vi "S4GUI.vi"(7 "Tab ObsEng":enum32{"Obs", "CCD modes", "Eng"}(tab)) -> ()   [LabVIEW 2018] (continued)
            n3007 = call-dynamic "Write State Machine.vi"("error in (no error)"=w6568, "State Machine.lvclass"=w6572, "Device in"=w6570) -> ("error out"=w6574:errorcluster, "Device out"=w6573:refnum<class "Channel.lvclass">)  [unwired: 7 in]
            n3008 = call-dynamic "Write Channel.vi"("error in (no error)"=w6574, "Channel.lvclass"=w6573, "Acquisition in"=w6566) -> ("error out"=w6562:errorcluster, "Acquisition out"=w6563:refnum<class "Acquisition.lvclass">)  [unwired: 7 in]
          }
        }
        n3009 = case shown="True" w6446 {
          tunnel: w6448 -> [w6490 w6522]
          tunnel: w6447 -> [w6489 w6521]
          tunnel: [w6490 w6520] -> w6469
          tunnel: [w6489 w6519] -> w6468
          tunnel: w6459 -> [_ w6502]
          tunnel: w6433 -> [_ w6501]
          tunnel: w6434 -> [_ w6500]
          tunnel: w6427 -> [_ w6499]
          tunnel: w6432 -> [_ w6498]
          tunnel: w6431 -> [_ w6493]
          frame False {
          }
          frame True {
            (unwired) 12 ("State")
            n3010 = call-dynamic "Read Channel.vi"("error in (no error)"=w6521, "Acquisition in"=w6522) -> ("error out"=w6496:errorcluster, "Channel.lvclass"=w6497:refnum<class "Channel.lvclass">, "Acquisition out"=w6531:refnum<class "Acquisition.lvclass">)  [unwired: 7 in]
            n3011 = local read "Filter4"() -> (w6503:u8)
            n3012 = call-dynamic "Write Filter.vi"("error in (no error)"=w6496, "Filter"=w6503, "Channel in"=w6497) -> ("error out"=w6518:errorcluster, "Channel out"=w6507:refnum<class "Channel.lvclass">)  [unwired: 7 in]
            n3013 = call-dynamic "Read Interface.vi"("error in (no error)"=w6518, "Channel in"=w6507) -> ("error out"=w6517:errorcluster, "Interface.lvclass"=w6516:refnum<class "Interface.lvclass">, "Channel out"=w6506:refnum<class "Channel.lvclass">)  [unwired: 7 in]
            n3014 = call-dynamic "Write Suffix.vi"("error in (no error)"=w6517, "Suffix"=w6502, "Interface in"=w6516) -> ("error out"=w6508:errorcluster, "Interface out"=w6511:refnum<class "Interface.lvclass">)  [unwired: 7 in]
            n3015 = call-dynamic "Write ObsType.vi"("error in (no error)"=w6508, "ObsType"=w6501, "Interface in"=w6511) -> ("error out"=w6509:errorcluster, "Interface out"=w6512:refnum<class "Interface.lvclass">)  [unwired: 7 in]
            n3016 = call-dynamic "Write Object.vi"("error in (no error)"=w6509, "Object"=w6500, "Interface in"=w6512) -> ("error out"=w6510:errorcluster, "Interface out"=w6513:refnum<class "Interface.lvclass">)  [unwired: 7 in]
            n3017 = call-dynamic "Write Comments.vi"("error in (no error)"=w6510, "Comments"=w6499, "Interface in"=w6513) -> ("error out"=w6514:errorcluster, "Interface out"=w6515:refnum<class "Interface.lvclass">)  [unwired: 7 in]
            n3018 = call-dynamic "Write Observer.vi"("error in (no error)"=w6514, "Observer"=w6498, "Interface in"=w6515) -> ("error out"=w6495:errorcluster, "Interface out"=w6494:refnum<class "Interface.lvclass">)  [unwired: 7 in]
            n3019 = call-dynamic "Write Project ID.vi"("error in (no error)"=w6495, "Project ID"=w6493, "Interface in"=w6494) -> ("error out"=w6491:errorcluster, "Interface out"=w6492:refnum<class "Interface.lvclass">)  [unwired: 7 in]
            n3020 = call-dynamic "Write Interface.vi"("error in (no error)"=w6491, "Interface.lvclass"=w6492, "Channel in"=w6506) -> ("error out"=w6504:errorcluster, "Channel out"=w6505:refnum<class "Channel.lvclass">)  [unwired: 7 in]
            n3021 = call-dynamic "Read State Machine.vi"("error in (no error)"=w6504, "Device in"=w6505) -> ("error out"=w6530:errorcluster, "State Machine.lvclass"=w6526:refnum<class "State Machine.lvclass">, "Device out"=w6527:refnum<class "Channel.lvclass">)  [unwired: 7 in]
            n3022 = call-dynamic "Write State.vi"("error in (no error)"=w6530, "State"=300, "State Machine in"=w6526) -> ("error out"=w6529:errorcluster, "State Machine out"=w6525:refnum<class "State Machine.lvclass">)  [unwired: 7 in]
            n3023 = call-dynamic "Write State Machine.vi"("error in (no error)"=w6529, "State Machine.lvclass"=w6525, "Device in"=w6527) -> ("error out"=w6523:errorcluster, "Device out"=w6524:refnum<class "Channel.lvclass">)  [unwired: 7 in]
            n3024 = call-dynamic "Write Channel.vi"("error in (no error)"=w6523, "Channel.lvclass"=w6524, "Acquisition in"=w6531) -> ("error out"=w6519:errorcluster, "Acquisition out"=w6520:refnum<class "Acquisition.lvclass">)  [unwired: 7 in]
          }
        }
        n3025 = call-dynamic "Write AcquisitionA.vi"("error in (no error)"=w6486, "Acquisition.lvclass"=w6487, "S4ACS_GUI in"=w6488) -> ("error out"=w6476:errorcluster, "S4ACS_GUI out"=w6480:refnum<class "S4GUI.lvclass">)  [unwired: 7 in]
        n3026 = call "Write AcquisitionB.vi"("error in (no error)"=w6481, "Acquisition.lvclass"=w6482, "S4ACS_GUI in"=w6480) -> ("error out"=w6475:errorcluster, "S4ACS_GUI out"=w6479:refnum<class "S4GUI.lvclass">)  [unwired: 7 in]
        n3027 = call-dynamic "Write AcquisitionC.vi"("error in (no error)"=w6470, "Acquisition.lvclass"=w6471, "S4ACS_GUI in"=w6479) -> ("error out"=w6474:errorcluster, "S4ACS_GUI out"=w6478:refnum<class "S4GUI.lvclass">)  [unwired: 7 in]
        n3028 = call-dynamic "Write AcquisitionD.vi"("error in (no error)"=w6468, "Acquisition.lvclass"=w6469, "S4ACS_GUI in"=w6478) -> ("error out"=w6473:errorcluster, "S4ACS_GUI out"=w6477:refnum<class "S4GUI.lvclass">)  [unwired: 7 in]
        n3029 = Merge Errors(w6476, w6475, w6474, w6473) -> (w6472:errorcluster)
        n3030 = call "Write cfg file.vi"("error in (no error)"=w6472, "cfg file"="lastsaved.cfg", "S4ACS_GUI in"=w6477) -> ("error out"=w6484:errorcluster, "S4ACS_GUI out"=w6483:refnum<class "S4GUI.lvclass">)  [unwired: 7 in]
      }
      event "Object_sflat", "Object_dark", "Object_zero", "Object_dflat", "Object_focus", "Object_obj": Value Change {
        n3031 = event-data() -> ("NewVal"=w6686:string)  [unwired: 1 in, 5 out]
        n3032 = stacked-sequence {
          seq-local: [w6716 _ _ _] -> [_ w6780 _ _]
          seq-local: [w6715 _ _ _] -> [_ w6779 _ _]
          seq-local: [_ w6778 _ _] -> [_ _ w6829 _]
          seq-local: [_ w6777 _ _] -> [_ _ w6828 _]
          seq-local: [_ _ w6827 _] -> [_ _ _ w6878]
          seq-local: [_ _ w6826 _] -> [_ _ _ w6877]
          tunnel: w6693 -> [w6728 _ _ _]
          tunnel: w6694 -> [w6727 _ _ _]
          tunnel: [_ _ _ w6876] -> w6688
          tunnel: [_ _ _ w6875] -> w6687
          tunnel: w6692 -> [w6714 w6776 w6825 w6874]
          tunnel: w6691 -> [w6713 w6775 w6811 w6860]
          tunnel: w6689 -> [w6712 w6761 w6810 w6859]
          tunnel: w6686 -> [w6711 w6760 w6809 w6858]
          tunnel: w6690 -> [w6710 w6759 w6808 w6857]
          frame #0 {
            # "observer"
            # "comment"
            # "object"
            # "suffix"
            # "obsType"
            n3033 = call-dynamic "Read AcquisitionA.vi"("error in (no error)"=w6728, "S4ACS_GUI in"=w6727) -> ("error out"=w6726:errorcluster, "Acquisition.lvclass"=w6725:refnum<class "Acquisition.lvclass">, "S4ACS_GUI out"=w6720:refnum<class "S4GUI.lvclass">)  [unwired: 7 in]
            n3034 = call-dynamic "Read Channel.vi"("error in (no error)"=w6726, "Acquisition in"=w6725) -> ("error out"=w6696:errorcluster, "Channel.lvclass"=w6699:refnum<class "Channel.lvclass">, "Acquisition out"=w6719:refnum<class "Acquisition.lvclass">)  [unwired: 7 in]
            n3035 = local read "Filter1"() -> (w6697:u8)
            n3036 = call-dynamic "Write Filter.vi"("error in (no error)"=w6696, "Filter"=w6697, "Channel in"=w6699) -> ("error out"=w6695:errorcluster, "Channel out"=w6698:refnum<class "Channel.lvclass">)  [unwired: 7 in]
            n3037 = call-dynamic "Read Interface.vi"("error in (no error)"=w6695, "Channel in"=w6698) -> ("error out"=w6706:errorcluster, "Interface.lvclass"=w6707:refnum<class "Interface.lvclass">, "Channel out"=w6724:refnum<class "Channel.lvclass">)  [unwired: 7 in]
            n3038 = call-dynamic "Write Suffix.vi"("error in (no error)"=w6706, "Suffix"=w6714, "Interface in"=w6707) -> ("error out"=w6731:errorcluster, "Interface out"=w6723:refnum<class "Interface.lvclass">)  [unwired: 7 in]
            n3039 = call-dynamic "Write ObsType.vi"("error in (no error)"=w6731, "ObsType"=w6712, "Interface in"=w6723) -> ("error out"=w6730:errorcluster, "Interface out"=w6722:refnum<class "Interface.lvclass">)  [unwired: 7 in]
            n3040 = call-dynamic "Write Object.vi"("error in (no error)"=w6730, "Object"=w6711, "Interface in"=w6722) -> ("error out"=w6729:errorcluster, "Interface out"=w6721:refnum<class "Interface.lvclass">)  [unwired: 7 in]
            n3041 = call-dynamic "Write Comments.vi"("error in (no error)"=w6729, "Comments"=w6713, "Interface in"=w6721) -> ("error out"=w6709:errorcluster, "Interface out"=w6708:refnum<class "Interface.lvclass">)  [unwired: 7 in]
            n3042 = call-dynamic "Write Observer.vi"("error in (no error)"=w6709, "Observer"=w6710, "Interface in"=w6708) -> ("error out"=w6704:errorcluster, "Interface out"=w6705:refnum<class "Interface.lvclass">)  [unwired: 7 in]
            n3043 = call-dynamic "Write Interface.vi"("error in (no error)"=w6704, "Interface.lvclass"=w6705, "Channel in"=w6724) -> ("error out"=w6701:errorcluster, "Channel out"=w6703:refnum<class "Channel.lvclass">)  [unwired: 7 in]
            n3044 = disable-structure shown="Enabled" {
              disable-tunnel: w6703 -> [w6741 w6743]
              disable-tunnel: [w6739 w6743] -> w6702
              disable-tunnel: w6701 -> [w6738 w6742]
              disable-tunnel: [w6733 w6742] -> w6700
              frame Disabled {
                n3045 = call-dynamic "Read State Machine.vi"("error in (no error)"=w6738, "Device in"=w6741) -> ("error out"=w6737:errorcluster, "State Machine.lvclass"=w6735:refnum<class "State Machine.lvclass">, "Device out"=w6740:refnum<class "Channel.lvclass">)  [unwired: 7 in]
                n3046 = call "Next State.vi"("error in (no error)"=w6737, "New_State"=12, "State Machine in"=w6735) -> ("error out"=w6736:errorcluster, "State Machine out"=w6734:refnum<class "State Machine.lvclass">)  [unwired: 7 in]
                n3047 = call-dynamic "Write State Machine.vi"("error in (no error)"=w6736, "State Machine.lvclass"=w6734, "Device in"=w6740) -> ("error out"=w6733:errorcluster, "Device out"=w6739:refnum<class "Channel.lvclass">)  [unwired: 7 in]
              }
              frame Enabled {
              }
            }
            n3048 = call-dynamic "Write Channel.vi"("error in (no error)"=w6700, "Channel.lvclass"=w6702, "Acquisition in"=w6719) -> ("error out"=w6717:errorcluster, "Acquisition out"=w6718:refnum<class "Acquisition.lvclass">)  [unwired: 7 in]
            n3049 = call-dynamic "Write AcquisitionA.vi"("error in (no error)"=w6717, "Acquisition.lvclass"=w6718, "S4ACS_GUI in"=w6720) -> ("error out"=w6715:errorcluster, "S4ACS_GUI out"=w6716:refnum<class "S4GUI.lvclass">)  [unwired: 7 in]
          }
          frame #1 {
            # "object"
            # "suffix"
            # "obsType"
            n3050 = call "Read AcquisitionB.vi"("error in (no error)"=w6779, "S4ACS_GUI in"=w6780) -> ("error out"=w6765:errorcluster, "Acquisition.lvclass"=w6766:refnum<class "Acquisition.lvclass">, "S4ACS_GUI out"=w6771:refnum<class "S4GUI.lvclass">)  [unwired: 7 in]
            n3051 = call-dynamic "Read Channel.vi"("error in (no error)"=w6765, "Acquisition in"=w6766) -> ("error out"=w6745:errorcluster, "Channel.lvclass"=w6747:refnum<class "Channel.lvclass">, "Acquisition out"=w6772:refnum<class "Acquisition.lvclass">)  [unwired: 7 in]
            n3052 = local read "Filter2"() -> (w6748:u8)
            n3053 = call-dynamic "Write Filter.vi"("error in (no error)"=w6745, "Filter"=w6748, "Channel in"=w6747) -> ("error out"=w6744:errorcluster, "Channel out"=w6746:refnum<class "Channel.lvclass">)  [unwired: 7 in]
            n3054 = call-dynamic "Read Interface.vi"("error in (no error)"=w6744, "Channel in"=w6746) -> ("error out"=w6753:errorcluster, "Interface.lvclass"=w6754:refnum<class "Interface.lvclass">, "Channel out"=w6767:refnum<class "Channel.lvclass">)  [unwired: 7 in]
            n3055 = call-dynamic "Write Suffix.vi"("error in (no error)"=w6753, "Suffix"=w6776, "Interface in"=w6754) -> ("error out"=w6762:errorcluster, "Interface out"=w6768:refnum<class "Interface.lvclass">)  [unwired: 7 in]
            n3056 = call-dynamic "Write ObsType.vi"("error in (no error)"=w6762, "ObsType"=w6761, "Interface in"=w6768) -> ("error out"=w6763:errorcluster, "Interface out"=w6769:refnum<class "Interface.lvclass">)  [unwired: 7 in]
            n3057 = call-dynamic "Write Object.vi"("error in (no error)"=w6763, "Object"=w6760, "Interface in"=w6769) -> ("error out"=w6764:errorcluster, "Interface out"=w6770:refnum<class "Interface.lvclass">)  [unwired: 7 in]
            n3058 = call-dynamic "Write Comments.vi"("error in (no error)"=w6764, "Comments"=w6775, "Interface in"=w6770) -> ("error out"=w6756:errorcluster, "Interface out"=w6755:refnum<class "Interface.lvclass">)  [unwired: 7 in]
            n3059 = call-dynamic "Write Observer.vi"("error in (no error)"=w6756, "Observer"=w6759, "Interface in"=w6755) -> ("error out"=w6757:errorcluster, "Interface out"=w6758:refnum<class "Interface.lvclass">)  [unwired: 7 in]
            n3060 = call-dynamic "Write Interface.vi"("error in (no error)"=w6757, "Interface.lvclass"=w6758, "Channel in"=w6767) -> ("error out"=w6751:errorcluster, "Channel out"=w6752:refnum<class "Channel.lvclass">)  [unwired: 7 in]
            n3061 = disable-structure shown="Enabled" {
              disable-tunnel: w6752 -> [w6785 w6792]
              disable-tunnel: w6751 -> [w6784 w6791]
              disable-tunnel: [w6782 w6792] -> w6750
              disable-tunnel: [w6781 w6791] -> w6749
              frame Disabled {
                n3062 = call-dynamic "Read State Machine.vi"("error in (no error)"=w6784, "Device in"=w6785) -> ("error out"=w6790:errorcluster, "State Machine.lvclass"=w6788:refnum<class "State Machine.lvclass">, "Device out"=w6783:refnum<class "Channel.lvclass">)  [unwired: 7 in]
                n3063 = call "Next State.vi"("error in (no error)"=w6790, "New_State"=12, "State Machine in"=w6788) -> ("error out"=w6789:errorcluster, "State Machine out"=w6787:refnum<class "State Machine.lvclass">)  [unwired: 7 in]
                n3064 = call-dynamic "Write State Machine.vi"("error in (no error)"=w6789, "State Machine.lvclass"=w6787, "Device in"=w6783) -> ("error out"=w6781:errorcluster, "Device out"=w6782:refnum<class "Channel.lvclass">)  [unwired: 7 in]
              }
              frame Enabled {
              }
            }
            n3065 = call-dynamic "Write Channel.vi"("error in (no error)"=w6749, "Channel.lvclass"=w6750, "Acquisition in"=w6772) -> ("error out"=w6774:errorcluster, "Acquisition out"=w6773:refnum<class "Acquisition.lvclass">)  [unwired: 7 in]
            n3066 = call "Write AcquisitionB.vi"("error in (no error)"=w6774, "Acquisition.lvclass"=w6773, "S4ACS_GUI in"=w6771) -> ("error out"=w6777:errorcluster, "S4ACS_GUI out"=w6778:refnum<class "S4GUI.lvclass">)  [unwired: 7 in]
          }
          frame #2 {
            # "object"
            # "suffix"
            # "obsType"
            n3067 = call-dynamic "Read AcquisitionC.vi"("error in (no error)"=w6828, "S4ACS_GUI in"=w6829) -> ("error out"=w6821:errorcluster, "Acquisition.lvclass"=w6820:refnum<class "Acquisition.lvclass">, "S4ACS_GUI out"=w6815:refnum<class "S4GUI.lvclass">)  [unwired: 7 in]
            n3068 = call-dynamic "Read Channel.vi"("error in (no error)"=w6821, "Acquisition in"=w6820) -> ("error out"=w6794:errorcluster, "Channel.lvclass"=w6796:refnum<class "Channel.lvclass">, "Acquisition out"=w6814:refnum<class "Acquisition.lvclass">)  [unwired: 7 in]
            n3069 = local read "Filter3"() -> (w6797:u8)
            n3070 = call-dynamic "Write Filter.vi"("error in (no error)"=w6794, "Filter"=w6797, "Channel in"=w6796) -> ("error out"=w6793:errorcluster, "Channel out"=w6795:refnum<class "Channel.lvclass">)  [unwired: 7 in]
            n3071 = call-dynamic "Read Interface.vi"("error in (no error)"=w6793, "Channel in"=w6795) -> ("error out"=w6806:errorcluster, "Interface.lvclass"=w6807:refnum<class "Interface.lvclass">, "Channel out"=w6819:refnum<class "Channel.lvclass">)  [unwired: 7 in]
            n3072 = call-dynamic "Write Suffix.vi"("error in (no error)"=w6806, "Suffix"=w6825, "Interface in"=w6807) -> ("error out"=w6824:errorcluster, "Interface out"=w6818:refnum<class "Interface.lvclass">)  [unwired: 7 in]
            n3073 = call-dynamic "Write ObsType.vi"("error in (no error)"=w6824, "ObsType"=w6810, "Interface in"=w6818) -> ("error out"=w6823:errorcluster, "Interface out"=w6817:refnum<class "Interface.lvclass">)  [unwired: 7 in]
            n3074 = call-dynamic "Write Object.vi"("error in (no error)"=w6823, "Object"=w6809, "Interface in"=w6817) -> ("error out"=w6822:errorcluster, "Interface out"=w6816:refnum<class "Interface.lvclass">)  [unwired: 7 in]
            n3075 = call-dynamic "Write Comments.vi"("error in (no error)"=w6822, "Comments"=w6811, "Interface in"=w6816) -> ("error out"=w6803:errorcluster, "Interface out"=w6802:refnum<class "Interface.lvclass">)  [unwired: 7 in]
            n3076 = call-dynamic "Write Observer.vi"("error in (no error)"=w6803, "Observer"=w6808, "Interface in"=w6802) -> ("error out"=w6804:errorcluster, "Interface out"=w6805:refnum<class "Interface.lvclass">)  [unwired: 7 in]
            n3077 = call-dynamic "Write Interface.vi"("error in (no error)"=w6804, "Interface.lvclass"=w6805, "Channel in"=w6819) -> ("error out"=w6800:errorcluster, "Channel out"=w6801:refnum<class "Channel.lvclass">)  [unwired: 7 in]
            n3078 = disable-structure shown="Enabled" {
              disable-tunnel: w6801 -> [w6836 w6841]
              disable-tunnel: w6800 -> [w6835 w6840]
              disable-tunnel: [w6833 w6841] -> w6799
              disable-tunnel: [w6830 w6840] -> w6798
              frame Disabled {
                n3079 = call-dynamic "Read State Machine.vi"("error in (no error)"=w6835, "Device in"=w6836) -> ("error out"=w6839:errorcluster, "State Machine.lvclass"=w6832:refnum<class "State Machine.lvclass">, "Device out"=w6834:refnum<class "Channel.lvclass">)  [unwired: 7 in]
                n3080 = call "Next State.vi"("error in (no error)"=w6839, "New_State"=12, "State Machine in"=w6832) -> ("error out"=w6838:errorcluster, "State Machine out"=w6831:refnum<class "State Machine.lvclass">)  [unwired: 7 in]
                n3081 = call-dynamic "Write State Machine.vi"("error in (no error)"=w6838, "State Machine.lvclass"=w6831, "Device in"=w6834) -> ("error out"=w6830:errorcluster, "Device out"=w6833:refnum<class "Channel.lvclass">)  [unwired: 7 in]
              }
              frame Enabled {
              }
            }
            n3082 = call-dynamic "Write Channel.vi"("error in (no error)"=w6798, "Channel.lvclass"=w6799, "Acquisition in"=w6814) -> ("error out"=w6812:errorcluster, "Acquisition out"=w6813:refnum<class "Acquisition.lvclass">)  [unwired: 7 in]
            n3083 = call-dynamic "Write AcquisitionC.vi"("error in (no error)"=w6812, "Acquisition.lvclass"=w6813, "S4ACS_GUI in"=w6815) -> ("error out"=w6826:errorcluster, "S4ACS_GUI out"=w6827:refnum<class "S4GUI.lvclass">)  [unwired: 7 in]
          }
          frame #3 {
            # "object"
            # "suffix"
            # "obsType"
            n3084 = call-dynamic "Read AcquisitionD.vi"("error in (no error)"=w6877, "S4ACS_GUI in"=w6878) -> ("error out"=w6870:errorcluster, "Acquisition.lvclass"=w6869:refnum<class "Acquisition.lvclass">, "S4ACS_GUI out"=w6864:refnum<class "S4GUI.lvclass">)  [unwired: 7 in]
            n3085 = call-dynamic "Read Channel.vi"("error in (no error)"=w6870, "Acquisition in"=w6869) -> ("error out"=w6843:errorcluster, "Channel.lvclass"=w6845:refnum<class "Channel.lvclass">, "Acquisition out"=w6863:refnum<class "Acquisition.lvclass">)  [unwired: 7 in]
            n3086 = local read "Filter4"() -> (w6846:u8)
            n3087 = call-dynamic "Write Filter.vi"("error in (no error)"=w6843, "Filter"=w6846, "Channel in"=w6845) -> ("error out"=w6842:errorcluster, "Channel out"=w6844:refnum<class "Channel.lvclass">)  [unwired: 7 in]
            n3088 = call-dynamic "Read Interface.vi"("error in (no error)"=w6842, "Channel in"=w6844) -> ("error out"=w6855:errorcluster, "Interface.lvclass"=w6856:refnum<class "Interface.lvclass">, "Channel out"=w6868:refnum<class "Channel.lvclass">)  [unwired: 7 in]
            n3089 = call-dynamic "Write Suffix.vi"("error in (no error)"=w6855, "Suffix"=w6874, "Interface in"=w6856) -> ("error out"=w6873:errorcluster, "Interface out"=w6867:refnum<class "Interface.lvclass">)  [unwired: 7 in]
            n3090 = call-dynamic "Write ObsType.vi"("error in (no error)"=w6873, "ObsType"=w6859, "Interface in"=w6867) -> ("error out"=w6872:errorcluster, "Interface out"=w6866:refnum<class "Interface.lvclass">)  [unwired: 7 in]
            n3091 = call-dynamic "Write Object.vi"("error in (no error)"=w6872, "Object"=w6858, "Interface in"=w6866) -> ("error out"=w6871:errorcluster, "Interface out"=w6865:refnum<class "Interface.lvclass">)  [unwired: 7 in]
            n3092 = call-dynamic "Write Comments.vi"("error in (no error)"=w6871, "Comments"=w6860, "Interface in"=w6865) -> ("error out"=w6854:errorcluster, "Interface out"=w6853:refnum<class "Interface.lvclass">)  [unwired: 7 in]
            n3093 = call-dynamic "Write Observer.vi"("error in (no error)"=w6854, "Observer"=w6857, "Interface in"=w6853) -> ("error out"=w6852:errorcluster, "Interface out"=w6851:refnum<class "Interface.lvclass">)  [unwired: 7 in]
            n3094 = call-dynamic "Write Interface.vi"("error in (no error)"=w6852, "Interface.lvclass"=w6851, "Channel in"=w6868) -> ("error out"=w6848:errorcluster, "Channel out"=w6850:refnum<class "Channel.lvclass">)  [unwired: 7 in]
            n3095 = disable-structure shown="Enabled" {
              disable-tunnel: w6850 -> [w6885 w6890]
              disable-tunnel: [w6883 w6890] -> w6849
              disable-tunnel: w6848 -> [w6882 w6889]
              disable-tunnel: [w6881 w6889] -> w6847
              frame Disabled {
                n3096 = call-dynamic "Read State Machine.vi"("error in (no error)"=w6882, "Device in"=w6885) -> ("error out"=w6888:errorcluster, "State Machine.lvclass"=w6880:refnum<class "State Machine.lvclass">, "Device out"=w6884:refnum<class "Channel.lvclass">)  [unwired: 7 in]
                n3097 = call "Next State.vi"("error in (no error)"=w6888, "New_State"=12, "State Machine in"=w6880) -> ("error out"=w6887:errorcluster, "State Machine out"=w6879:refnum<class "State Machine.lvclass">)  [unwired: 7 in]
                n3098 = call-dynamic "Write State Machine.vi"("error in (no error)"=w6887, "State Machine.lvclass"=w6879, "Device in"=w6884) -> ("error out"=w6881:errorcluster, "Device out"=w6883:refnum<class "Channel.lvclass">)  [unwired: 7 in]
              }
              frame Enabled {
              }
            }
            n3099 = call-dynamic "Write Channel.vi"("error in (no error)"=w6847, "Channel.lvclass"=w6849, "Acquisition in"=w6863) -> ("error out"=w6861:errorcluster, "Acquisition out"=w6862:refnum<class "Acquisition.lvclass">)  [unwired: 7 in]
            n3100 = call-dynamic "Write AcquisitionD.vi"("error in (no error)"=w6861, "Acquisition.lvclass"=w6862, "S4ACS_GUI in"=w6864) -> ("error out"=w6875:errorcluster, "S4ACS_GUI out"=w6876:refnum<class "S4GUI.lvclass">)  [unwired: 7 in]
          }
        }
      }
      event "DFLAT Comments", "SFLAT Comments", "DARK Comments", "ZERO Comments", "FOCUS Comments", "OBJECT Comments": Value Change {
        n3101 = event-data() -> ("NewVal"=w6891:string)  [unwired: 1 in, 5 out]
        n3102 = disable-structure shown="Enabled" {
          disable-tunnel: w6899 -> [w6908 w7082]
          disable-tunnel: w6898 -> [w6907 w7081]
          disable-tunnel: w6897 -> [w6906 _]
          disable-tunnel: w6896 -> [w6905 _]
          disable-tunnel: w6895 -> [w6904 _]
          disable-tunnel: w6894 -> [w6903 _]
          disable-tunnel: [w6902 w7082] -> w6893
          disable-tunnel: [w6901 w7081] -> w6892
          disable-tunnel: w6891 -> [w6900 _]
          frame Disabled {
            n3103 = stacked-sequence {
              seq-local: [w6936 _ _ _] -> [_ w6994 _ _]
              seq-local: [w6935 _ _ _] -> [_ w6993 _ _]
              seq-local: [_ w6992 _ _] -> [_ _ w7037 _]
              seq-local: [_ w6991 _ _] -> [_ _ w7036 _]
              seq-local: [_ _ w7035 _] -> [_ _ _ w7080]
              seq-local: [_ _ w7034 _] -> [_ _ _ w7079]
              tunnel: w6907 -> [w6948 _ _ _]
              tunnel: w6908 -> [w6947 _ _ _]
              tunnel: [_ _ _ w7078] -> w6902
              tunnel: [_ _ _ w7077] -> w6901
              tunnel: w6905 -> [w6934 w6990 w7033 w7076]
              tunnel: w6900 -> [w6933 w6989 w7019 w7062]
              tunnel: w6903 -> [w6932 w6975 w7018 w7061]
              tunnel: w6906 -> [w6931 w6974 w7017 w7060]
              tunnel: w6904 -> [w6930 w6973 w7016 w7059]
              frame #0 {
                # "observer"
                # "comment"
                # "object"
                # "suffix"
                # "obsType"
                n3104 = call-dynamic "Read AcquisitionA.vi"("error in (no error)"=w6948, "S4ACS_GUI in"=w6947) -> ("error out"=w6946:errorcluster, "Acquisition.lvclass"=w6945:refnum<class "Acquisition.lvclass">, "S4ACS_GUI out"=w6940:refnum<class "S4GUI.lvclass">)  [unwired: 7 in]
                n3105 = call-dynamic "Read Channel.vi"("error in (no error)"=w6946, "Acquisition in"=w6945) -> ("error out"=w6910:errorcluster, "Channel.lvclass"=w6913:refnum<class "Channel.lvclass">, "Acquisition out"=w6939:refnum<class "Acquisition.lvclass">)  [unwired: 7 in]
                n3106 = local read "Filter1"() -> (w6911:u8)
                n3107 = call-dynamic "Write Filter.vi"("error in (no error)"=w6910, "Filter"=w6911, "Channel in"=w6913) -> ("error out"=w6909:errorcluster, "Channel out"=w6912:refnum<class "Channel.lvclass">)  [unwired: 7 in]
                n3108 = call-dynamic "Read Interface.vi"("error in (no error)"=w6909, "Channel in"=w6912) -> ("error out"=w6926:errorcluster, "Interface.lvclass"=w6927:refnum<class "Interface.lvclass">, "Channel out"=w6944:refnum<class "Channel.lvclass">)  [unwired: 7 in]
                n3109 = call-dynamic "Write Suffix.vi"("error in (no error)"=w6926, "Suffix"=w6934, "Interface in"=w6927) -> ("error out"=w6951:errorcluster, "Interface out"=w6943:refnum<class "Interface.lvclass">)  [unwired: 7 in]
                n3110 = call-dynamic "Write ObsType.vi"("error in (no error)"=w6951, "ObsType"=w6932, "Interface in"=w6943) -> ("error out"=w6950:errorcluster, "Interface out"=w6942:refnum<class "Interface.lvclass">)  [unwired: 7 in]
                n3111 = call-dynamic "Write Object.vi"("error in (no error)"=w6950, "Object"=w6931, "Interface in"=w6942) -> ("error out"=w6949:errorcluster, "Interface out"=w6941:refnum<class "Interface.lvclass">)  [unwired: 7 in]
                n3112 = call-dynamic "Write Comments.vi"("error in (no error)"=w6949, "Comments"=w6933, "Interface in"=w6941) -> ("error out"=w6929:errorcluster, "Interface out"=w6928:refnum<class "Interface.lvclass">)  [unwired: 7 in]
                n3113 = call-dynamic "Write Observer.vi"("error in (no error)"=w6929, "Observer"=w6930, "Interface in"=w6928) -> ("error out"=w6924:errorcluster, "Interface out"=w6925:refnum<class "Interface.lvclass">)  [unwired: 7 in]
                n3114 = call-dynamic "Write Interface.vi"("error in (no error)"=w6924, "Interface.lvclass"=w6925, "Channel in"=w6944) -> ("error out"=w6920:errorcluster, "Channel out"=w6923:refnum<class "Channel.lvclass">)  [unwired: 7 in]
                n3115 = call-dynamic "Read State Machine.vi"("error in (no error)"=w6920, "Device in"=w6923) -> ("error out"=w6919:errorcluster, "State Machine.lvclass"=w6917:refnum<class "State Machine.lvclass">, "Device out"=w6922:refnum<class "Channel.lvclass">)  [unwired: 7 in]
                n3116 = call "Next State.vi"("error in (no error)"=w6919, "New_State"=12, "State Machine in"=w6917) -> ("error out"=w6918:errorcluster, "State Machine out"=w6916:refnum<class "State Machine.lvclass">)  [unwired: 7 in]
                n3117 = call-dynamic "Write State Machine.vi"("error in (no error)"=w6918, "State Machine.lvclass"=w6916, "Device in"=w6922) -> ("error out"=w6915:errorcluster, "Device out"=w6921:refnum<class "Channel.lvclass">)  [unwired: 7 in]
                n3118 = call-dynamic "Write Channel.vi"("error in (no error)"=w6915, "Channel.lvclass"=w6921, "Acquisition in"=w6939) -> ("error out"=w6937:errorcluster, "Acquisition out"=w6938:refnum<class "Acquisition.lvclass">)  [unwired: 7 in]
                n3119 = call-dynamic "Write AcquisitionA.vi"("error in (no error)"=w6937, "Acquisition.lvclass"=w6938, "S4ACS_GUI in"=w6940) -> ("error out"=w6935:errorcluster, "S4ACS_GUI out"=w6936:refnum<class "S4GUI.lvclass">)  [unwired: 7 in]
              }
              frame #1 {
                # "object"
                # "suffix"
                # "obsType"
                n3120 = call "Read AcquisitionB.vi"("error in (no error)"=w6993, "S4ACS_GUI in"=w6994) -> ("error out"=w6979:errorcluster, "Acquisition.lvclass"=w6980:refnum<class "Acquisition.lvclass">, "S4ACS_GUI out"=w6985:refnum<class "S4GUI.lvclass">)  [unwired: 7 in]
                n3121 = call-dynamic "Read Channel.vi"("error in (no error)"=w6979, "Acquisition in"=w6980) -> ("error out"=w6953:errorcluster, "Channel.lvclass"=w6955:refnum<class "Channel.lvclass">, "Acquisition out"=w6986:refnum<class "Acquisition.lvclass">)  [unwired: 7 in]
                n3122 = local read "Filter2"() -> (w6956:u8)
                n3123 = call-dynamic "Write Filter.vi"("error in (no error)"=w6953, "Filter"=w6956, "Channel in"=w6955) -> ("error out"=w6952:errorcluster, "Channel out"=w6954:refnum<class "Channel.lvclass">)  [unwired: 7 in]
                n3124 = call-dynamic "Read Interface.vi"("error in (no error)"=w6952, "Channel in"=w6954) -> ("error out"=w6967:errorcluster, "Interface.lvclass"=w6968:refnum<class "Interface.lvclass">, "Channel out"=w6981:refnum<class "Channel.lvclass">)  [unwired: 7 in]
                n3125 = call-dynamic "Write Suffix.vi"("error in (no error)"=w6967, "Suffix"=w6990, "Interface in"=w6968) -> ("error out"=w6976:errorcluster, "Interface out"=w6982:refnum<class "Interface.lvclass">)  [unwired: 7 in]
                n3126 = call-dynamic "Write ObsType.vi"("error in (no error)"=w6976, "ObsType"=w6975, "Interface in"=w6982) -> ("error out"=w6977:errorcluster, "Interface out"=w6983:refnum<class "Interface.lvclass">)  [unwired: 7 in]
                n3127 = call-dynamic "Write Object.vi"("error in (no error)"=w6977, "Object"=w6974, "Interface in"=w6983) -> ("error out"=w6978:errorcluster, "Interface out"=w6984:refnum<class "Interface.lvclass">)  [unwired: 7 in]
                n3128 = call-dynamic "Write Comments.vi"("error in (no error)"=w6978, "Comments"=w6989, "Interface in"=w6984) -> ("error out"=w6970:errorcluster, "Interface out"=w6969:refnum<class "Interface.lvclass">)  [unwired: 7 in]
                n3129 = call-dynamic "Write Observer.vi"("error in (no error)"=w6970, "Observer"=w6973, "Interface in"=w6969) -> ("error out"=w6971:errorcluster, "Interface out"=w6972:refnum<class "Interface.lvclass">)  [unwired: 7 in]
                n3130 = call-dynamic "Write Interface.vi"("error in (no error)"=w6971, "Interface.lvclass"=w6972, "Channel in"=w6981) -> ("error out"=w6960:errorcluster, "Channel out"=w6961:refnum<class "Channel.lvclass">)  [unwired: 7 in]
                n3131 = call-dynamic "Read State Machine.vi"("error in (no error)"=w6960, "Device in"=w6961) -> ("error out"=w6966:errorcluster, "State Machine.lvclass"=w6964:refnum<class "State Machine.lvclass">, "Device out"=w6959:refnum<class "Channel.lvclass">)  [unwired: 7 in]
                n3132 = call "Next State.vi"("error in (no error)"=w6966, "New_State"=12, "State Machine in"=w6964) -> ("error out"=w6965:errorcluster, "State Machine out"=w6963:refnum<class "State Machine.lvclass">)  [unwired: 7 in]
                n3133 = call-dynamic "Write State Machine.vi"("error in (no error)"=w6965, "State Machine.lvclass"=w6963, "Device in"=w6959) -> ("error out"=w6957:errorcluster, "Device out"=w6958:refnum<class "Channel.lvclass">)  [unwired: 7 in]
                n3134 = call-dynamic "Write Channel.vi"("error in (no error)"=w6957, "Channel.lvclass"=w6958, "Acquisition in"=w6986) -> ("error out"=w6988:errorcluster, "Acquisition out"=w6987:refnum<class "Acquisition.lvclass">)  [unwired: 7 in]
                n3135 = call "Write AcquisitionB.vi"("error in (no error)"=w6988, "Acquisition.lvclass"=w6987, "S4ACS_GUI in"=w6985) -> ("error out"=w6991:errorcluster, "S4ACS_GUI out"=w6992:refnum<class "S4GUI.lvclass">)  [unwired: 7 in]
              }
              frame #2 {
                # "object"
                # "suffix"
                # "obsType"
                n3136 = call-dynamic "Read AcquisitionC.vi"("error in (no error)"=w7036, "S4ACS_GUI in"=w7037) -> ("error out"=w7029:errorcluster, "Acquisition.lvclass"=w7028:refnum<class "Acquisition.lvclass">, "S4ACS_GUI out"=w7023:refnum<class "S4GUI.lvclass">)  [unwired: 7 in]
                n3137 = call-dynamic "Read Channel.vi"("error in (no error)"=w7029, "Acquisition in"=w7028) -> ("error out"=w6996:errorcluster, "Channel.lvclass"=w6998:refnum<class "Channel.lvclass">, "Acquisition out"=w7022:refnum<class "Acquisition.lvclass">)  [unwired: 7 in]
                n3138 = local read "Filter3"() -> (w6999:u8)
                n3139 = call-dynamic "Write Filter.vi"("error in (no error)"=w6996, "Filter"=w6999, "Channel in"=w6998) -> ("error out"=w6995:errorcluster, "Channel out"=w6997:refnum<class "Channel.lvclass">)  [unwired: 7 in]
                n3140 = call-dynamic "Read Interface.vi"("error in (no error)"=w6995, "Channel in"=w6997) -> ("error out"=w7014:errorcluster, "Interface.lvclass"=w7015:refnum<class "Interface.lvclass">, "Channel out"=w7027:refnum<class "Channel.lvclass">)  [unwired: 7 in]
                n3141 = call-dynamic "Write Suffix.vi"("error in (no error)"=w7014, "Suffix"=w7033, "Interface in"=w7015) -> ("error out"=w7032:errorcluster, "Interface out"=w7026:refnum<class "Interface.lvclass">)  [unwired: 7 in]
                n3142 = call-dynamic "Write ObsType.vi"("error in (no error)"=w7032, "ObsType"=w7018, "Interface in"=w7026) -> ("error out"=w7031:errorcluster, "Interface out"=w7025:refnum<class "Interface.lvclass">)  [unwired: 7 in]
                n3143 = call-dynamic "Write Object.vi"("error in (no error)"=w7031, "Object"=w7017, "Interface in"=w7025) -> ("error out"=w7030:errorcluster, "Interface out"=w7024:refnum<class "Interface.lvclass">)  [unwired: 7 in]
                n3144 = call-dynamic "Write Comments.vi"("error in (no error)"=w7030, "Comments"=w7019, "Interface in"=w7024) -> ("error out"=w7011:errorcluster, "Interface out"=w7010:refnum<class "Interface.lvclass">)  [unwired: 7 in]
                n3145 = call-dynamic "Write Observer.vi"("error in (no error)"=w7011, "Observer"=w7016, "Interface in"=w7010) -> ("error out"=w7012:errorcluster, "Interface out"=w7013:refnum<class "Interface.lvclass">)  [unwired: 7 in]
                n3146 = call-dynamic "Write Interface.vi"("error in (no error)"=w7012, "Interface.lvclass"=w7013, "Channel in"=w7027) -> ("error out"=w7005:errorcluster, "Channel out"=w7006:refnum<class "Channel.lvclass">)  [unwired: 7 in]
                n3147 = call-dynamic "Read State Machine.vi"("error in (no error)"=w7005, "Device in"=w7006) -> ("error out"=w7009:errorcluster, "State Machine.lvclass"=w7002:refnum<class "State Machine.lvclass">, "Device out"=w7004:refnum<class "Channel.lvclass">)  [unwired: 7 in]
                n3148 = call "Next State.vi"("error in (no error)"=w7009, "New_State"=12, "State Machine in"=w7002) -> ("error out"=w7008:errorcluster, "State Machine out"=w7001:refnum<class "State Machine.lvclass">)  [unwired: 7 in]
                n3149 = call-dynamic "Write State Machine.vi"("error in (no error)"=w7008, "State Machine.lvclass"=w7001, "Device in"=w7004) -> ("error out"=w7000:errorcluster, "Device out"=w7003:refnum<class "Channel.lvclass">)  [unwired: 7 in]
                n3150 = call-dynamic "Write Channel.vi"("error in (no error)"=w7000, "Channel.lvclass"=w7003, "Acquisition in"=w7022) -> ("error out"=w7020:errorcluster, "Acquisition out"=w7021:refnum<class "Acquisition.lvclass">)  [unwired: 7 in]
                n3151 = call-dynamic "Write AcquisitionC.vi"("error in (no error)"=w7020, "Acquisition.lvclass"=w7021, "S4ACS_GUI in"=w7023) -> ("error out"=w7034:errorcluster, "S4ACS_GUI out"=w7035:refnum<class "S4GUI.lvclass">)  [unwired: 7 in]
              }
              frame #3 {
                # "object"
                # "suffix"
                # "obsType"
                n3152 = call-dynamic "Read AcquisitionD.vi"("error in (no error)"=w7079, "S4ACS_GUI in"=w7080) -> ("error out"=w7072:errorcluster, "Acquisition.lvclass"=w7071:refnum<class "Acquisition.lvclass">, "S4ACS_GUI out"=w7066:refnum<class "S4GUI.lvclass">)  [unwired: 7 in]
                n3153 = call-dynamic "Read Channel.vi"("error in (no error)"=w7072, "Acquisition in"=w7071) -> ("error out"=w7039:errorcluster, "Channel.lvclass"=w7041:refnum<class "Channel.lvclass">, "Acquisition out"=w7065:refnum<class "Acquisition.lvclass">)  [unwired: 7 in]
                n3154 = local read "Filter4"() -> (w7042:u8)
                n3155 = call-dynamic "Write Filter.vi"("error in (no error)"=w7039, "Filter"=w7042, "Channel in"=w7041) -> ("error out"=w7038:errorcluster, "Channel out"=w7040:refnum<class "Channel.lvclass">)  [unwired: 7 in]
                n3156 = call-dynamic "Read Interface.vi"("error in (no error)"=w7038, "Channel in"=w7040) -> ("error out"=w7057:errorcluster, "Interface.lvclass"=w7058:refnum<class "Interface.lvclass">, "Channel out"=w7070:refnum<class "Channel.lvclass">)  [unwired: 7 in]
                n3157 = call-dynamic "Write Suffix.vi"("error in (no error)"=w7057, "Suffix"=w7076, "Interface in"=w7058) -> ("error out"=w7075:errorcluster, "Interface out"=w7069:refnum<class "Interface.lvclass">)  [unwired: 7 in]
                n3158 = call-dynamic "Write ObsType.vi"("error in (no error)"=w7075, "ObsType"=w7061, "Interface in"=w7069) -> ("error out"=w7074:errorcluster, "Interface out"=w7068:refnum<class "Interface.lvclass">)  [unwired: 7 in]
                n3159 = call-dynamic "Write Object.vi"("error in (no error)"=w7074, "Object"=w7060, "Interface in"=w7068) -> ("error out"=w7073:errorcluster, "Interface out"=w7067:refnum<class "Interface.lvclass">)  [unwired: 7 in]
                n3160 = call-dynamic "Write Comments.vi"("error in (no error)"=w7073, "Comments"=w7062, "Interface in"=w7067) -> ("error out"=w7056:errorcluster, "Interface out"=w7055:refnum<class "Interface.lvclass">)  [unwired: 7 in]
                n3161 = call-dynamic "Write Observer.vi"("error in (no error)"=w7056, "Observer"=w7059, "Interface in"=w7055) -> ("error out"=w7051:errorcluster, "Interface out"=w7050:refnum<class "Interface.lvclass">)  [unwired: 7 in]
                n3162 = call-dynamic "Write Interface.vi"("error in (no error)"=w7051, "Interface.lvclass"=w7050, "Channel in"=w7070) -> ("error out"=w7046:errorcluster, "Channel out"=w7049:refnum<class "Channel.lvclass">)  [unwired: 7 in]
                n3163 = call-dynamic "Read State Machine.vi"("error in (no error)"=w7046, "Device in"=w7049) -> ("error out"=w7054:errorcluster, "State Machine.lvclass"=w7044:refnum<class "State Machine.lvclass">, "Device out"=w7048:refnum<class "Channel.lvclass">)  [unwired: 7 in]
                n3164 = call "Next State.vi"("error in (no error)"=w7054, "New_State"=12, "State Machine in"=w7044) -> ("error out"=w7053:errorcluster, "State Machine out"=w7043:refnum<class "State Machine.lvclass">)  [unwired: 7 in]
                n3165 = call-dynamic "Write State Machine.vi"("error in (no error)"=w7053, "State Machine.lvclass"=w7043, "Device in"=w7048) -> ("error out"=w7045:errorcluster, "Device out"=w7047:refnum<class "Channel.lvclass">)  [unwired: 7 in]
                n3166 = call-dynamic "Write Channel.vi"("error in (no error)"=w7045, "Channel.lvclass"=w7047, "Acquisition in"=w7065) -> ("error out"=w7063:errorcluster, "Acquisition out"=w7064:refnum<class "Acquisition.lvclass">)  [unwired: 7 in]
                n3167 = call-dynamic "Write AcquisitionD.vi"("error in (no error)"=w7063, "Acquisition.lvclass"=w7064, "S4ACS_GUI in"=w7066) -> ("error out"=w7077:errorcluster, "S4ACS_GUI out"=w7078:refnum<class "S4GUI.lvclass">)  [unwired: 7 in]
              }
            }
          }
          frame Enabled {
          }
        }
      }
      event "object suffix", "dflat suffix", "sflat suffix", "dark suffix", "zero suffix", "focus suffix": Value Change {
        # "Remove todos <\\n> e <space> do sufixo:"
        n3168 = event-data() -> ("NewVal"=w7092:string)  [unwired: 1 in, 5 out]
        n3169 = To Lower Case(string=w7092) -> (all lower case string=w7091:string)
        n3170 = call <vilib>:"Trim Whitespace.vi"("string"=w7091) -> ("trimmed string"=w7090:string)  [unwired: 1 in]
        n3171 = Search and Replace String(replace all?=TRUE ("replace all? (F)"), input string=w7090, search string="\n") -> (result string=w7089:string)  [unwired: 5 in, 3 out]
        n3172 = call <vilib>:"Space Constant.vi"() -> ("String"=w7087:string)
        n3173 = Search and Replace String(replace all?=TRUE ("replace all? (F)"), input string=w7089, search string=w7087) -> (result string=w7083:string)  [unwired: 5 in, 3 out]
        n3174 = case shown="\"FOCUS\"" w7084 {
          tunnel: w7083 -> [w7101 w7102 w7103 w7104 w7105 w7106]
          frame "OBJECT", Default {
            n3175 = local write "object suffix"(w7101) -> ()
          }
          frame "DFLAT" {
            n3176 = local write "dflat suffix"(w7102) -> ()
          }
          frame "SFLAT" {
            n3177 = local write "sflat suffix"(w7103) -> ()
          }
          frame "DARK" {
            n3178 = local write "dark suffix"(w7104) -> ()
          }
          frame "ZERO" {
            n3179 = local write "zero suffix"(w7105) -> ()
          }
          frame "FOCUS" {
            n3180 = local write "focus suffix"(w7106) -> ()
          }
        }
        n3181 = stacked-sequence {
          seq-local: [w7128 _ _ _] -> [_ w7192 _ _]
          seq-local: [w7127 _ _ _] -> [_ w7191 _ _]
          seq-local: [_ w7190 _ _] -> [_ _ w7241 _]
          seq-local: [_ w7189 _ _] -> [_ _ w7240 _]
          seq-local: [_ _ w7239 _] -> [_ _ _ w7290]
          seq-local: [_ _ w7238 _] -> [_ _ _ w7289]
          tunnel: w7099 -> [w7140 _ _ _]
          tunnel: w7100 -> [w7139 _ _ _]
          tunnel: [_ _ _ w7288] -> w7094
          tunnel: [_ _ _ w7287] -> w7093
          tunnel: w7083 -> [w7126 w7188 w7237 w7286]
          tunnel: w7097 -> [w7125 w7187 w7223 w7272]
          tunnel: w7095 -> [w7124 w7173 w7222 w7271]
          tunnel: w7098 -> [w7123 w7172 w7221 w7270]
          tunnel: w7096 -> [w7122 w7171 w7220 w7269]
          frame #0 {
            # "observer"
            # "comment"
            # "object"
            # "suffix"
            # "obsType"
            n3182 = call-dynamic "Read AcquisitionA.vi"("error in (no error)"=w7140, "S4ACS_GUI in"=w7139) -> ("error out"=w7138:errorcluster, "Acquisition.lvclass"=w7137:refnum<class "Acquisition.lvclass">, "S4ACS_GUI out"=w7132:refnum<class "S4GUI.lvclass">)  [unwired: 7 in]
            n3183 = call-dynamic "Read Channel.vi"("error in (no error)"=w7138, "Acquisition in"=w7137) -> ("error out"=w7108:errorcluster, "Channel.lvclass"=w7111:refnum<class "Channel.lvclass">, "Acquisition out"=w7131:refnum<class "Acquisition.lvclass">)  [unwired: 7 in]
            n3184 = local read "Filter1"() -> (w7109:u8)
            n3185 = call-dynamic "Write Filter.vi"("error in (no error)"=w7108, "Filter"=w7109, "Channel in"=w7111) -> ("error out"=w7107:errorcluster, "Channel out"=w7110:refnum<class "Channel.lvclass">)  [unwired: 7 in]
            n3186 = call-dynamic "Read Interface.vi"("error in (no error)"=w7107, "Channel in"=w7110) -> ("error out"=w7118:errorcluster, "Interface.lvclass"=w7119:refnum<class "Interface.lvclass">, "Channel out"=w7136:refnum<class "Channel.lvclass">)  [unwired: 7 in]
            n3187 = call-dynamic "Write Suffix.vi"("error in (no error)"=w7118, "Suffix"=w7126, "Interface in"=w7119) -> ("error out"=w7143:errorcluster, "Interface out"=w7135:refnum<class "Interface.lvclass">)  [unwired: 7 in]
            n3188 = call-dynamic "Write ObsType.vi"("error in (no error)"=w7143, "ObsType"=w7124, "Interface in"=w7135) -> ("error out"=w7142:errorcluster, "Interface out"=w7134:refnum<class "Interface.lvclass">)  [unwired: 7 in]
            n3189 = call-dynamic "Write Object.vi"("error in (no error)"=w7142, "Object"=w7123, "Interface in"=w7134) -> ("error out"=w7141:errorcluster, "Interface out"=w7133:refnum<class "Interface.lvclass">)  [unwired: 7 in]
            n3190 = call-dynamic "Write Comments.vi"("error in (no error)"=w7141, "Comments"=w7125, "Interface in"=w7133) -> ("error out"=w7121:errorcluster, "Interface out"=w7120:refnum<class "Interface.lvclass">)  [unwired: 7 in]
            n3191 = call-dynamic "Write Observer.vi"("error in (no error)"=w7121, "Observer"=w7122, "Interface in"=w7120) -> ("error out"=w7116:errorcluster, "Interface out"=w7117:refnum<class "Interface.lvclass">)  [unwired: 7 in]
            n3192 = call-dynamic "Write Interface.vi"("error in (no error)"=w7116, "Interface.lvclass"=w7117, "Channel in"=w7136) -> ("error out"=w7113:errorcluster, "Channel out"=w7115:refnum<class "Channel.lvclass">)  [unwired: 7 in]
            n3193 = disable-structure shown="Enabled" {
              disable-tunnel: w7115 -> [w7153 w7155]
              disable-tunnel: [w7151 w7155] -> w7114
              disable-tunnel: w7113 -> [w7150 w7154]
              disable-tunnel: [w7145 w7154] -> w7112
              frame Disabled {
                n3194 = call-dynamic "Read State Machine.vi"("error in (no error)"=w7150, "Device in"=w7153) -> ("error out"=w7149:errorcluster, "State Machine.lvclass"=w7147:refnum<class "State Machine.lvclass">, "Device out"=w7152:refnum<class "Channel.lvclass">)  [unwired: 7 in]
                n3195 = call "Next State.vi"("error in (no error)"=w7149, "New_State"=12, "State Machine in"=w7147) -> ("error out"=w7148:errorcluster, "State Machine out"=w7146:refnum<class "State Machine.lvclass">)  [unwired: 7 in]
                n3196 = call-dynamic "Write State Machine.vi"("error in (no error)"=w7148, "State Machine.lvclass"=w7146, "Device in"=w7152) -> ("error out"=w7145:errorcluster, "Device out"=w7151:refnum<class "Channel.lvclass">)  [unwired: 7 in]
              }
              frame Enabled {
              }
            }
            n3197 = call-dynamic "Write Channel.vi"("error in (no error)"=w7112, "Channel.lvclass"=w7114, "Acquisition in"=w7131) -> ("error out"=w7129:errorcluster, "Acquisition out"=w7130:refnum<class "Acquisition.lvclass">)  [unwired: 7 in]
            n3198 = call-dynamic "Write AcquisitionA.vi"("error in (no error)"=w7129, "Acquisition.lvclass"=w7130, "S4ACS_GUI in"=w7132) -> ("error out"=w7127:errorcluster, "S4ACS_GUI out"=w7128:refnum<class "S4GUI.lvclass">)  [unwired: 7 in]
          }
          frame #1 {
            # "object"
            # "suffix"
            # "obsType"
            n3199 = call "Read AcquisitionB.vi"("error in (no error)"=w7191, "S4ACS_GUI in"=w7192) -> ("error out"=w7177:errorcluster, "Acquisition.lvclass"=w7178:refnum<class "Acquisition.lvclass">, "S4ACS_GUI out"=w7183:refnum<class "S4GUI.lvclass">)  [unwired: 7 in]
            n3200 = call-dynamic "Read Channel.vi"("error in (no error)"=w7177, "Acquisition in"=w7178) -> ("error out"=w7157:errorcluster, "Channel.lvclass"=w7159:refnum<class "Channel.lvclass">, "Acquisition out"=w7184:refnum<class "Acquisition.lvclass">)  [unwired: 7 in]
            n3201 = local read "Filter2"() -> (w7160:u8)
            n3202 = call-dynamic "Write Filter.vi"("error in (no error)"=w7157, "Filter"=w7160, "Channel in"=w7159) -> ("error out"=w7156:errorcluster, "Channel out"=w7158:refnum<class "Channel.lvclass">)  [unwired: 7 in]
            n3203 = call-dynamic "Read Interface.vi"("error in (no error)"=w7156, "Channel in"=w7158) -> ("error out"=w7165:errorcluster, "Interface.lvclass"=w7166:refnum<class "Interface.lvclass">, "Channel out"=w7179:refnum<class "Channel.lvclass">)  [unwired: 7 in]
            n3204 = call-dynamic "Write Suffix.vi"("error in (no error)"=w7165, "Suffix"=w7188, "Interface in"=w7166) -> ("error out"=w7174:errorcluster, "Interface out"=w7180:refnum<class "Interface.lvclass">)  [unwired: 7 in]
            n3205 = call-dynamic "Write ObsType.vi"("error in (no error)"=w7174, "ObsType"=w7173, "Interface in"=w7180) -> ("error out"=w7175:errorcluster, "Interface out"=w7181:refnum<class "Interface.lvclass">)  [unwired: 7 in]
            n3206 = call-dynamic "Write Object.vi"("error in (no error)"=w7175, "Object"=w7172, "Interface in"=w7181) -> ("error out"=w7176:errorcluster, "Interface out"=w7182:refnum<class "Interface.lvclass">)  [unwired: 7 in]
            n3207 = call-dynamic "Write Comments.vi"("error in (no error)"=w7176, "Comments"=w7187, "Interface in"=w7182) -> ("error out"=w7168:errorcluster, "Interface out"=w7167:refnum<class "Interface.lvclass">)  [unwired: 7 in]
            n3208 = call-dynamic "Write Observer.vi"("error in (no error)"=w7168, "Observer"=w7171, "Interface in"=w7167) -> ("error out"=w7169:errorcluster, "Interface out"=w7170:refnum<class "Interface.lvclass">)  [unwired: 7 in]
            n3209 = call-dynamic "Write Interface.vi"("error in (no error)"=w7169, "Interface.lvclass"=w7170, "Channel in"=w7179) -> ("error out"=w7163:errorcluster, "Channel out"=w7164:refnum<class "Channel.lvclass">)  [unwired: 7 in]
            n3210 = disable-structure shown="Enabled" {
              disable-tunnel: w7164 -> [w7197 w7204]
              disable-tunnel: w7163 -> [w7196 w7203]
              disable-tunnel: [w7194 w7204] -> w7162
              disable-tunnel: [w7193 w7203] -> w7161
              frame Disabled {
                n3211 = call-dynamic "Read State Machine.vi"("error in (no error)"=w7196, "Device in"=w7197) -> ("error out"=w7202:errorcluster, "State Machine.lvclass"=w7200:refnum<class "State Machine.lvclass">, "Device out"=w7195:refnum<class "Channel.lvclass">)  [unwired: 7 in]
                n3212 = call "Next State.vi"("error in (no error)"=w7202, "New_State"=12, "State Machine in"=w7200) -> ("error out"=w7201:errorcluster, "State Machine out"=w7199:refnum<class "State Machine.lvclass">)  [unwired: 7 in]
                n3213 = call-dynamic "Write State Machine.vi"("error in (no error)"=w7201, "State Machine.lvclass"=w7199, "Device in"=w7195) -> ("error out"=w7193:errorcluster, "Device out"=w7194:refnum<class "Channel.lvclass">)  [unwired: 7 in]
              }
              frame Enabled {
              }
            }
            n3214 = call-dynamic "Write Channel.vi"("error in (no error)"=w7161, "Channel.lvclass"=w7162, "Acquisition in"=w7184) -> ("error out"=w7186:errorcluster, "Acquisition out"=w7185:refnum<class "Acquisition.lvclass">)  [unwired: 7 in]
            n3215 = call "Write AcquisitionB.vi"("error in (no error)"=w7186, "Acquisition.lvclass"=w7185, "S4ACS_GUI in"=w7183) -> ("error out"=w7189:errorcluster, "S4ACS_GUI out"=w7190:refnum<class "S4GUI.lvclass">)  [unwired: 7 in]
          }
          frame #2 {
            # "object"
            # "suffix"
            # "obsType"
            n3216 = call-dynamic "Read AcquisitionC.vi"("error in (no error)"=w7240, "S4ACS_GUI in"=w7241) -> ("error out"=w7233:errorcluster, "Acquisition.lvclass"=w7232:refnum<class "Acquisition.lvclass">, "S4ACS_GUI out"=w7227:refnum<class "S4GUI.lvclass">)  [unwired: 7 in]
            n3217 = call-dynamic "Read Channel.vi"("error in (no error)"=w7233, "Acquisition in"=w7232) -> ("error out"=w7206:errorcluster, "Channel.lvclass"=w7208:refnum<class "Channel.lvclass">, "Acquisition out"=w7226:refnum<class "Acquisition.lvclass">)  [unwired: 7 in]
            n3218 = local read "Filter3"() -> (w7209:u8)
            n3219 = call-dynamic "Write Filter.vi"("error in (no error)"=w7206, "Filter"=w7209, "Channel in"=w7208) -> ("error out"=w7205:errorcluster, "Channel out"=w7207:refnum<class "Channel.lvclass">)  [unwired: 7 in]
            n3220 = call-dynamic "Read Interface.vi"("error in (no error)"=w7205, "Channel in"=w7207) -> ("error out"=w7218:errorcluster, "Interface.lvclass"=w7219:refnum<class "Interface.lvclass">, "Channel out"=w7231:refnum<class "Channel.lvclass">)  [unwired: 7 in]
            n3221 = call-dynamic "Write Suffix.vi"("error in (no error)"=w7218, "Suffix"=w7237, "Interface in"=w7219) -> ("error out"=w7236:errorcluster, "Interface out"=w7230:refnum<class "Interface.lvclass">)  [unwired: 7 in]
